vi "Assert Query Excuse Content.vi"() -> ()   [LabVIEW 2015, in "Admin_Actor.lvlib" / "ExcuseNotesHandler.lvclass"]
uses:
  ExcuseNotesHandler.lvclass
  API/_Database/Database.lvclass
  ExcuseNotesHandler.lvclass/ExcuseNotesHandler.ctl
panel:
  out "recordset data":variant[][](array[variant])
  in  "path":path=path "E:/哈工大竞技机器人队/机器人队管理系统/Database/CRTDatabase.accdb"
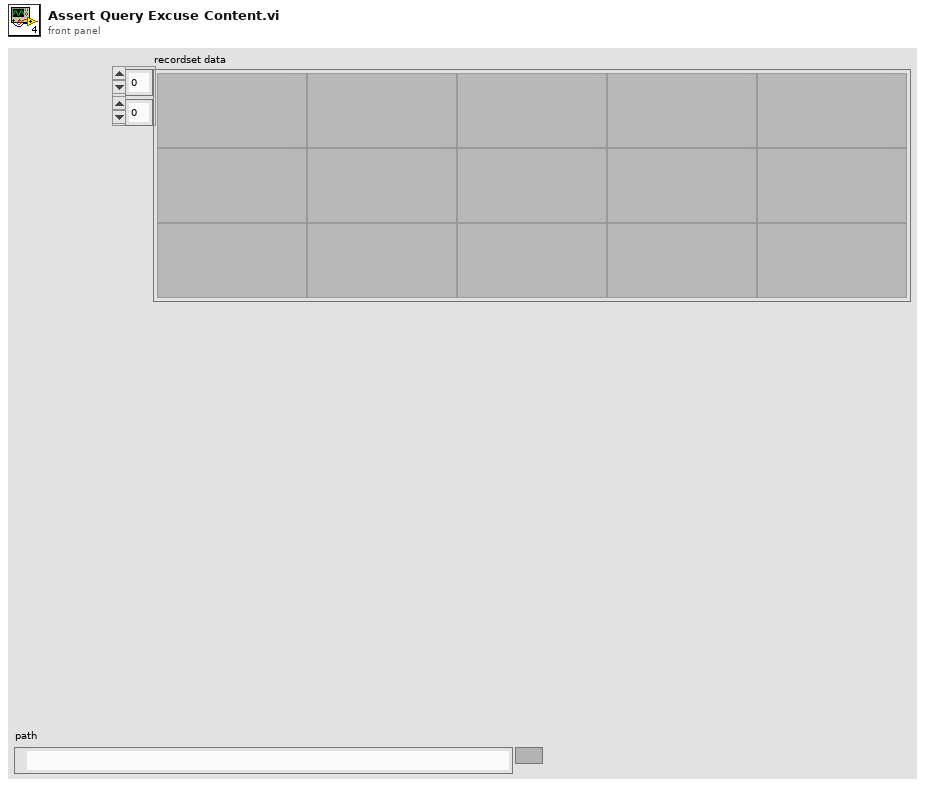
[diagram p1: front panel]
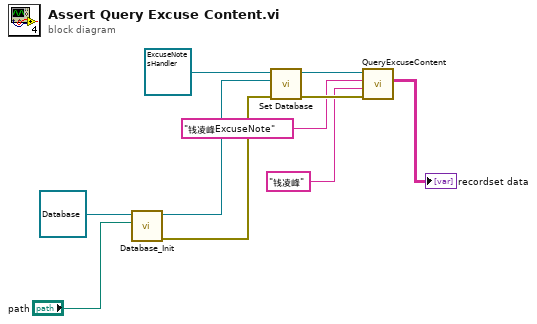
[diagram p0: block diagram]
diagram:
  n1 = call "Database_Init.vi"("path"="path", "object in"=refnum<class "Database.lvclass"> refnum ("Database")) -> ("error out"=w6:errorcluster, "object out"=w7:refnum<class "Database.lvclass">)  [unwired: 8 in]
  n2 = call "Set Database.vi"("error in (no error)"=w6, "Database"=w7, "ExcuseNotes in"=refnum<class "ExcuseNotesHandler.lvclass"> refnum ("Admin_Actor.lvlib:ExcuseNotes.lvclass")) -> ("error out"=w4:errorcluster, "ExcuseNotes out"=w5:refnum<class "ExcuseNotesHandler.lvclass">)  [unwired: 7 in]
  n3 = call "QueryExcuseContent.vi"("error in (no error)"=w4, "Name"="钱凌峰", "TableName"="钱凌峰ExcuseNote", "ExcuseNotes in"=w5) -> ("ExcuseNote(\"\")"=→"recordset data":string[][])  [unwired: 5 in, 2 out]
